vi "Pomiar_Wil_Temp.vi"() -> ()   [LabVIEW 2022 SP3]
uses:
  <vilib>/MakerHub/LINX/Public/Utilities/Open Serial.vi
  <vilib>/MakerHub/LINX/LMH-LINX.lvlib
panel:
  out "Temperature [°C]":u8(slide) scale=-10.0..40.0
  out "Humidity [%]":u8(knob) scale=0.1..100.0
  in  "?":bool
  in  "Serial Port":refnum<visa-resource-name>="N/A"
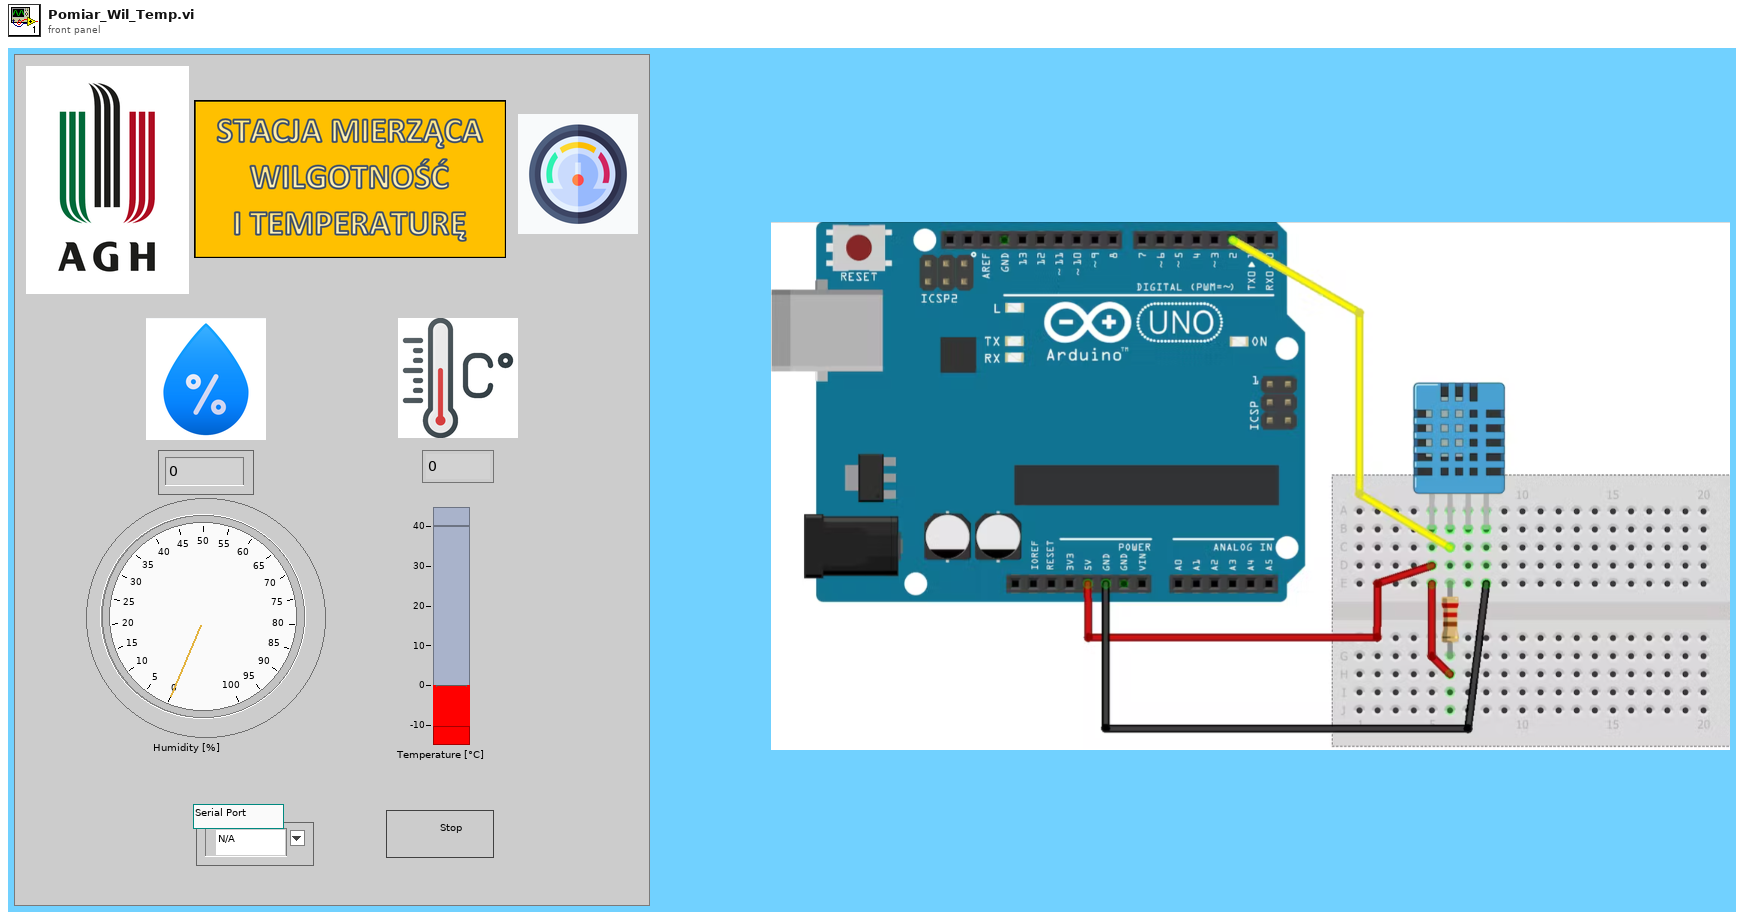
[diagram p1: front panel]
types:
  T1 = typedef "LMH-LINX.lvlib/LINX Ref.ctl" = cluster{"IO":T2, "Interface":T3, "LINX Device Config":T4}
  T2 = typedef "LMH-LINX.lvlib/Platform.ctl" = enum16{"Remote", "Local"}
  T3 = typedef "LMH-LINX.lvlib/Interface.ctl" = enum16{"Serial", "TCP"}
  T4 = typedef "LMH-LINX.lvlib/Device.lvlib/LINX Device Config.ctl" = cluster{"Interface":T3, "COM Port":refnum<visa-resource-name>, "TCP Configuration":T5, "Device Family":u8, "Device ID":u8, "Device Name":string, "TCP Ref":refnum<k5>, "Channels":T6}
  T5 = typedef "LMH-LINX.lvlib/Device.lvlib/TCP Config.ctl" = cluster{"IP Address":string, "Port":u16}
  T6 = typedef "LMH-LINX.lvlib/Channels.ctl" = cluster{"DI":u8[], "DO":u8[], "AI":u8[], "AO":u8[], "PWM":u8[], "QE":u8[], "UART":u8[], "I2C 2":u8[], "SPI":u8[], "CAN":u8[], "Servo":u8[], "AI Ref (V)":dbl, "AI Resolution (Bits)":u8, "AO Ref (V)":dbl, "AO Resolution (Bits)":u8}
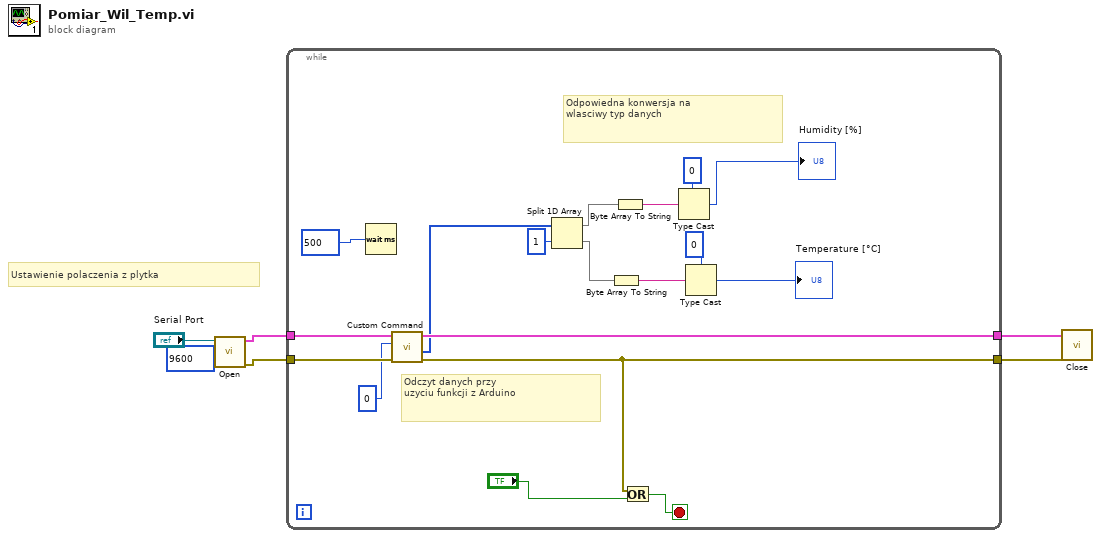
[diagram p0: block diagram]
diagram:
  # "Ustawienie polaczenia z plytka"
  n1 = call-poly <vilib>:"Open.vi"("Baud Rate Override"=u32 9600, "Serial Port"="Serial Port") -> ("Error Out"=w5:errorcluster, "LINX Resource"=w6:T1)  [unwired: 7 in, 1 out]
  n2 = while {
    tunnel: w6 -> [w24]
    tunnel: w5 -> [w23]
    tunnel: [w22] -> w4
    tunnel: [w20] -> w3
    stop <- w19 stop-if-true
    # "Odpowiedna konwersja na\nwlasciwy typ danych"
    # "Odczyt danych przy\nuzyciu funkcji z Arduino"
    n3 = Wait (ms)(milliseconds to wait=u32 500) -> ()  [unwired: 1 out]
    n4 = call <vilib>:"Custom Command.vi"("Error In"=w23, "Custom Command Number"=u16 0, "LINX Resource"=w24) -> ("Error Out"=w20:errorcluster, "Response"=w16:u8[], "LINX Resource"=w22:T1)  [unwired: 5 in, 1 out]
    n5 = Split 1D Array(array=w16, index=1) -> (first subarray=w14:u8[], second subarray=w13:u8[])
    n6 = Byte Array To String(unsigned byte array=w13) -> (string=w9:string)
    n7 = Byte Array To String(unsigned byte array=w14) -> (string=w11:string)
    n8 = Or(x=w20, y="?") -> (x .or. y?=w19:bool)
    n9 = Type Cast(type=u8 0, x=w11) -> (*(type *) &x=→"Humidity [%]":u8)
    n10 = Type Cast(type=u8 0, x=w9) -> (*(type *) &x=→"Temperature [°C]":u8)
  }
  n11 = call <vilib>:"Close.vi"("Error In"=w3, "LINX Resource"=w4) -> ()  [unwired: 9 in, 1 out]
